vi "specu1a 1.0.0 String to 8xU8 Cluster.vi"(13 "String in":string, 14 "offset (0)":i32) -> (2 "8xU8 Cluster":cluster{u8, u8, u8, u8, u8, u8, u8, u8})   [LabVIEW 2019]
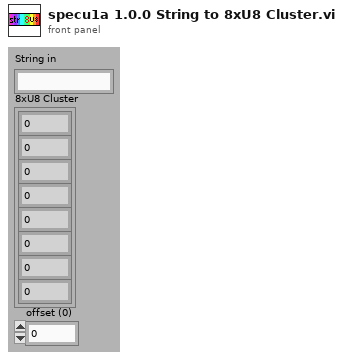
[diagram p1: front panel]
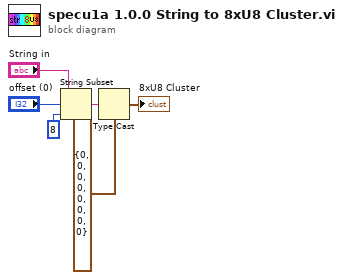
[diagram p0: block diagram]
diagram:
  n1 = String Subset(string="String in", offset (0)="offset (0)", length (rest)=8) -> (substring=w1:string)
  n2 = Type Cast(type=cluster{u8, u8, u8, u8, u8, u8, u8, u8} {0, 0, 0, 0, 0, 0, 0, 0}, x=w1) -> (*(type *) &x=→"8xU8 Cluster":cluster{u8, u8, u8, u8, u8, u8, u8, u8})
